vi "AverageOfArray.vi"(9 "Length of Sample":dbl, 10 "Start Index":dbl, 11 "Array In":dbl[](array[numeric])) -> (3 "Average":dbl)   [LabVIEW 2014]
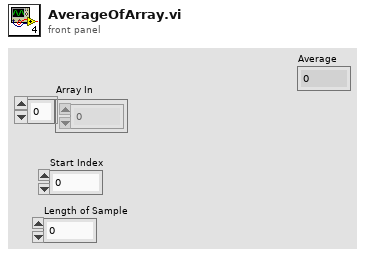
[diagram p1: front panel]
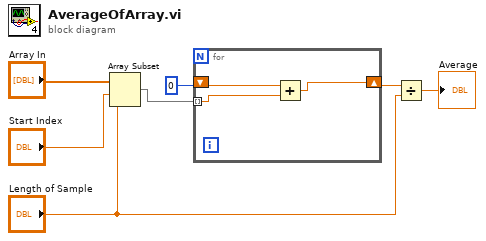
[diagram p0: block diagram]
diagram:
  n1 = Array Subset(array="Array In", index="Start Index", length="Length of Sample") -> (w4:dbl[])
  n2 = for {
    shift-right: [w8] -> w3
    shift-left: 0 -> [w10]
    tunnel: w4 -> [w9] mode=indexing
    n3 = Add(x=w10, y=w9) -> (x+y=w8:dbl)
  }
  n4 = Divide(x=w3, y="Length of Sample") -> (x/y=→"Average":dbl)
